vi "SiPM_Tests_Global_Var.vi"() -> ()   [LabVIEW 2019]
uses:
  <vilib>/Analysis/6fits.llb/Curve Fitting Criteria.ctl
  <vilib>/Analysis/NI_AALPro.lvlib
panel:
  in  "CH1 Trigger Logic":T1(ring)
  in  "CH1 Trigger Thr":dbl=0.003 caption="CH1 Trigger Thr (V)" step=0.001 format="%#_6p"
  out "CH3+CH4_spectrum":dbl[](array[numeric])
  in  "CH4 Trigger Logic":T1(ring)
  in  "CH4 Trigger":dbl caption="CH4 Trigger Thr (V)" step=0.001 format="%#_6p"
  in  "CH3 Trigger Logic":T1(ring)
  in  "CH3 Trigger":dbl caption="CH3 Trigger Thr (V)" step=0.001 format="%#_6p"
  in  "CH2 Trigger Logic":T1(ring)
  in  "CH2 Trigger thr":dbl caption="CH2 Trigger Thr (V)" step=0.001 format="%#_6p"
  out "Ch4_spectrum":dbl[](array[numeric])
  out "Ch3_Spectrum":dbl[](array[numeric])
  in  "Trigger Source":T2(ring)=enum."Channel 2"
  in  "Ch 2 V/Div":dbl(knob)=0.02 min=0.0 max=5.0 step=0.05 scale=0.0..5.0
  in  "Ch1 V/Div":dbl(knob)=0.02 min=0.0 max=5.0 step=0.001 scale=0.0..5.0
  in  "Keithley_V":dbl=30.0 format="%.3g"
  in  "Agilent_V":dbl=5.0 min=0.0 max=25.0 step=0.001 format="%.3g"
  in  "LE_Thr":dbl=0.127 caption="Leading Edge Thr" step=0.001 format="%#_6p"
  in  "Discriminator":bool
  in  "Integral/Peak":bool
  in  "Integral_Start":dbl
  in  "Integral_Stop":dbl
  in  "Disable Filtering":bool
  in  "Trigger Level":dbl(knob)=0.00213 min=-10.0 max=10.0 step=0.01 scale=0.0..5.0
  in  "Coincidence?":bool
  in  "Atten Nb Steps":u8=2 caption="Attenuation Nb of Steps" step=1
  in  "Attenuation Step":dbl=2.4 caption="Attenuation Step Size" step=0.1
  in  "Delay Nb Steps":u8=2 caption="Delay Nb of steps" step=1
  in  "Delay Step":dbl=2.4 caption="Delay Step Size (ns)" step=0.1
  in  "Threshold 2":dbl caption="Max_value" step=0.001 format="%#_6p"
  in  "Arduino Error":errorcluster
  in  "Arduino VISA":refnum<visa-resource-name>
  out "Y-Home":dbl
  out "X-Home":dbl
  out "Correction_factor":dbl[](array[numeric])
  in  "Threshold":dbl caption="Threshold (V)" step=0.001 format="%#_6p"
  out "Shifted_wvfrm":waveform(dbl)[](array[waveform])
  out "Ch2_spectrum":dbl[](array[numeric])
  out "Ch1_Spectrum":dbl[](array[numeric])
  in  "Wvfm Stop":i32=2 caption="Wvfm Stop (ns)"
  in  "Wvfm Start":i32=2 caption="Wvfm Start (ns)"
  in  "NbSamples":i64 caption="Nb of Samples to Analyze"
  in  "width":i32
  in  "threshold":dbl
  in  "method":T3=1 items=["Least Square", "Least Absolute Residual", "Bisquare"]
  in  "Init_std_dev":dbl=1.0
  in  "Offset":i64
  in  "Nb of Samples to Display":i32=50
  in  "TDMS file array":refnum<k34>[](array[refnum])
  in  "Waveform Nb":u16
  in  "Attenuation":dbl
  in  "Delay (ns)":dbl
  in  "Save Results?":bool
  out "Default?":bool
  out "App Dir":path
  in  "Directory":path=path "C:/Users/johnk/Desktop/ESA_Scintillator_Data"
  in  "File Name":string="1"
  in  "Hist Min":dbl format="%0.2f"
  in  "Hist Max":dbl format="%0.2f"
  out "Pulser VISA":refnum<visa-resource-name>
  out "Pulser Error":errorcluster
  out "PwrSupply VISA":refnum<visa-resource-name>
  out "PwrSupply Error":errorcluster
  out "Scope Error":errorcluster
  out "Scope VISA":refnum<visa-resource-name>
  in  "Session Log ref":refnum<vi>
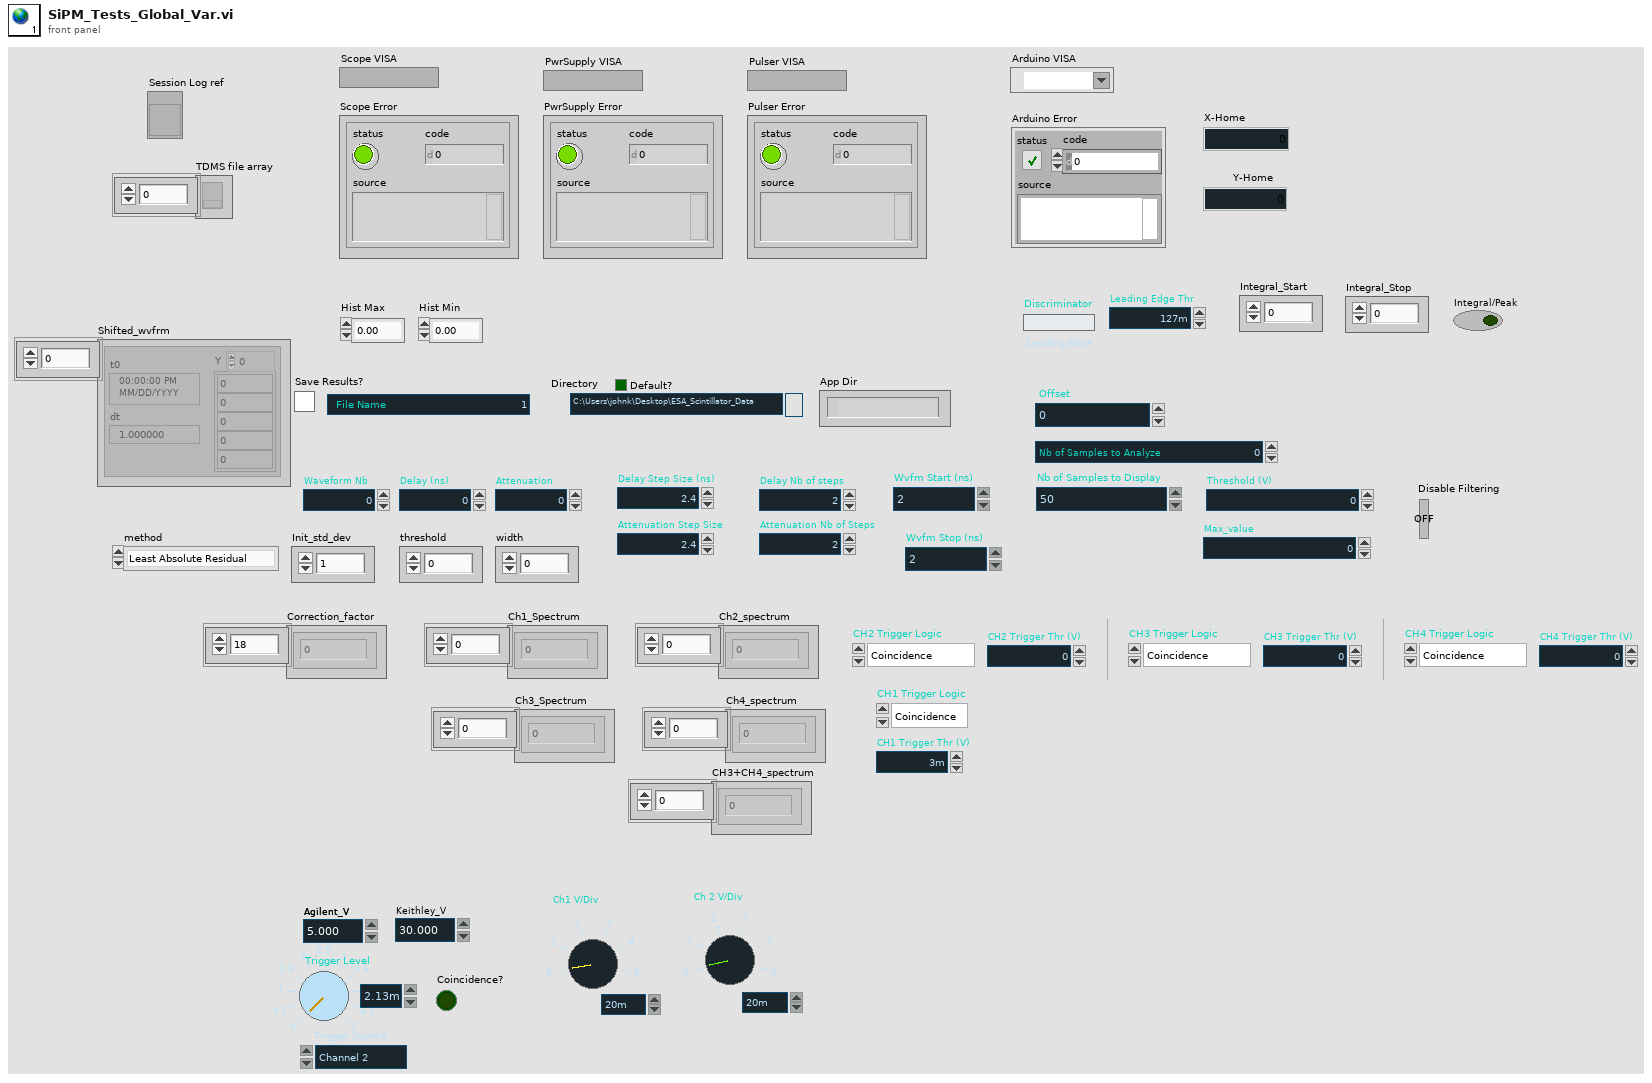
[diagram p1: front panel]
types:
  T1 = enum16{"Coincidence", "Anti-Coincidence", "Don't Care"}
  T2 = enum16{"Channel 1", "Channel 2", "Channel 3", "Channel 4", "D0", "D1", "D2", "D3", "D4", "D5", "D6", "D7", "D8", "D9", "D10", "D11", "D12", "D13", "D14", "D15", "External", "Power Line", "Waveform Generator"}
  T3 = typedef "NI_AALPro.lvlib/Curve Fitting Criteria.ctl" = u16
diagram:
